vi "NewtonsPSM_Conf_Power.vi"(0 "VISA session":refnum<visa-resource-name>, 7 "Integration (Signed)":u16(ring) items=["SIGNED", "MAGNITUDE"], 11 "error in (no error)":errorcluster) -> (4 "dup VISA session":refnum<visa-resource-name>, 15 "error out":errorcluster)   [LabVIEW 2025, in "NewtonsPSM1735.lvlib"]
doc: "This VI set the Power Meter parameters for the PPA2530."
uses:
  NewtonsPSM1735.lvlib
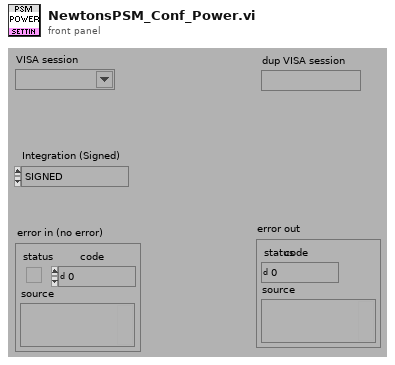
[diagram p1: front panel]
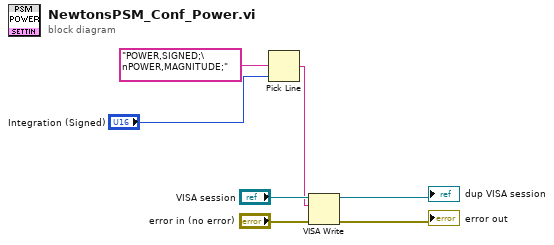
[diagram p0: block diagram]
diagram:
  n1 = Pick Line(multi-line string="POWER,SIGNED;\nPOWER,MAGNITUDE;", line index="Integration (Signed)") -> (output string=w2:string)  [unwired: 1 out]
  n2 = VISA Write(VISA resource name="VISA session", write buffer=w2, error in (no error)="error in (no error)") -> (VISA resource name out=→"dup VISA session":refnum<visa-resource-name>, error out=→"error out":errorcluster)  [unwired: 1 out]
